vi "Main.vi"() -> ()   [LabVIEW 2011]
uses:
  VendingStateCtr.ctl
panel:
  out "결과":string
  out "현재 잔액":i32
  in  "종료 버튼":bool
  in  "환불":bool
  in  "콜라 구입":bool
  in  "500원 투입":bool
  in  "100원 투입":bool
  in  "50원 투입":bool
  in  "Enum":T1
  # "동전 투입 버튼"
  # "자판기 기능 버튼"
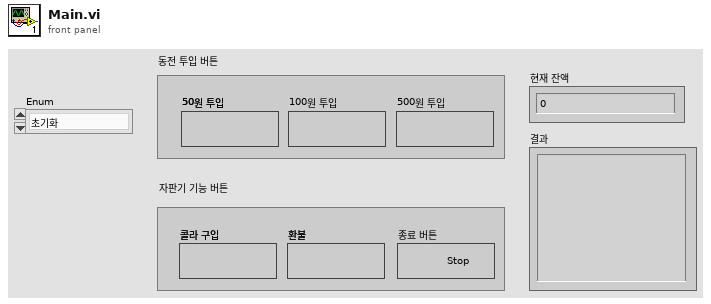
[diagram p1: front panel]
types:
  T1 = typedef "VendingStateCtr.ctl" = enum16{"초기화", "대기", "100원 투입", "500원 투입", "50원 투입", "판매", "환불", "종료"}
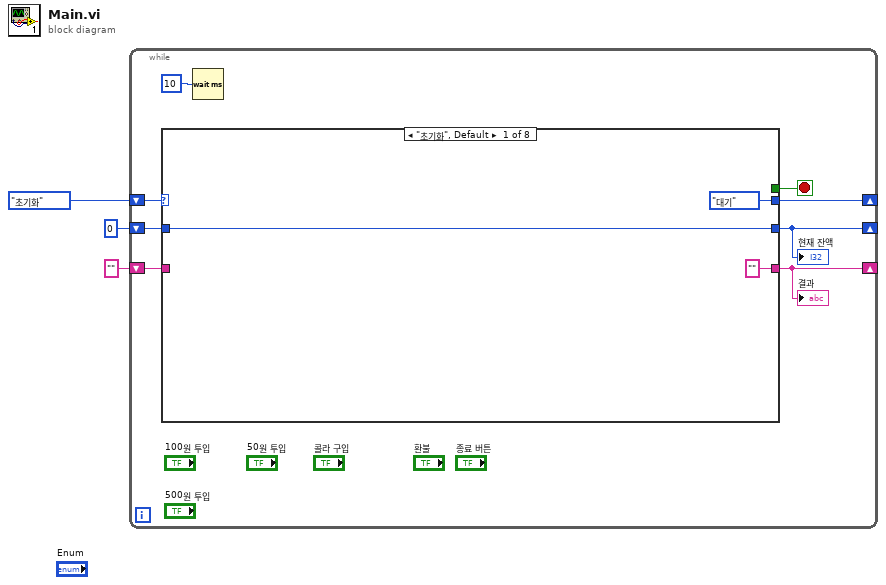
[diagram p0: block diagram]
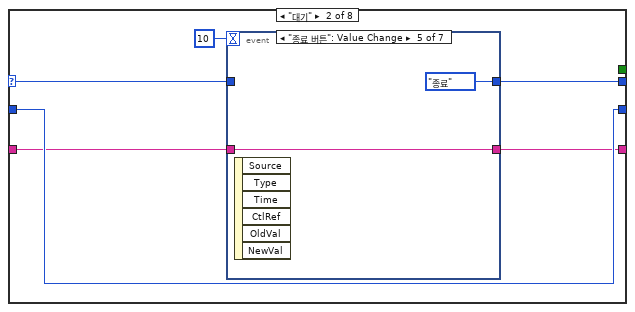
[diagram p2: hidden frame]
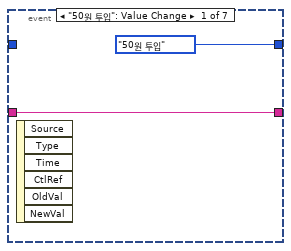
[diagram p3: hidden frame]
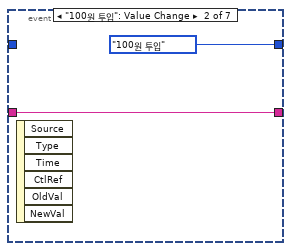
[diagram p4: hidden frame]
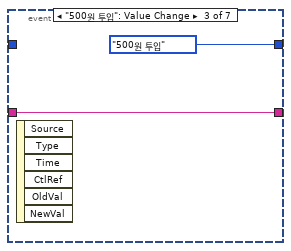
[diagram p5: hidden frame]
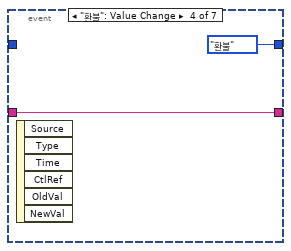
[diagram p6: hidden frame]
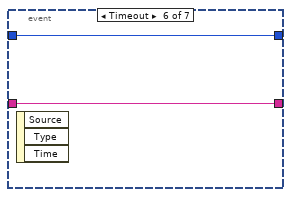
[diagram p7: hidden frame]
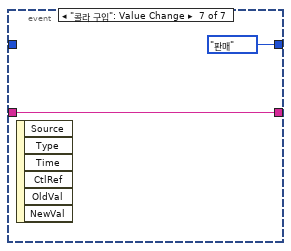
[diagram p8: hidden frame]
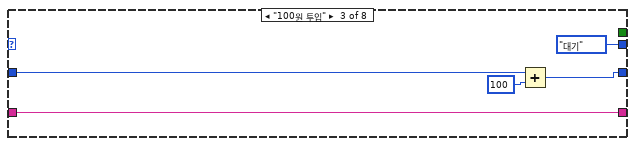
[diagram p9: hidden frame]
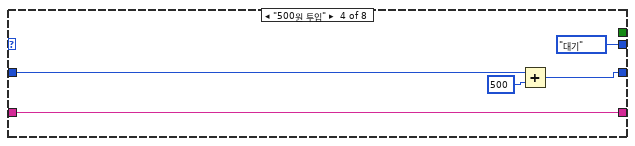
[diagram p10: hidden frame]
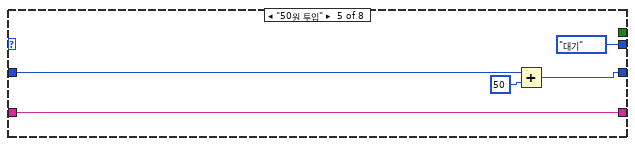
[diagram p11: hidden frame]
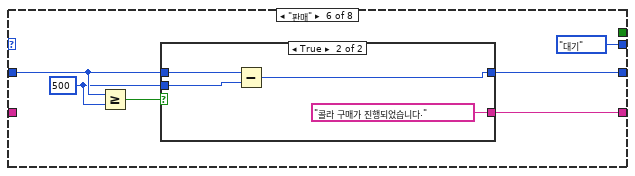
[diagram p12: hidden frame]
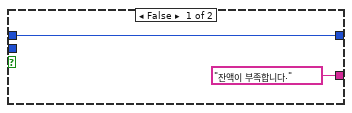
[diagram p13: hidden frame]
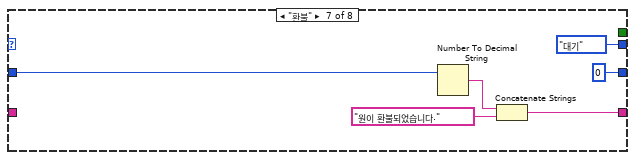
[diagram p14: hidden frame]
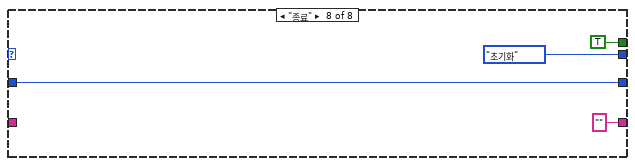
[diagram p15: hidden frame]
diagram:
  n1 = while {
    shift-right: [w9] -> _
    shift-left: VendingStateCtr."초기화" ("Enum") -> [w11]
    shift-right: [w7] -> _
    shift-left: 0 -> [w10]
    shift-right: [w4] -> _
    shift-left: "" -> [w5]
    stop <- w6 stop-if-true
    n2 = case shown="\"초기화\", Default" w11 {
      selector: w11 -> [_ w15 _ _ _ _ _ _]
      tunnel: w10 -> [w14 w18 w39 w44 w49 w52 w67 w70]
      tunnel: [w14 w18 w37 w42 w47 w51 0 w70] -> w7
      tunnel: [VendingStateCtr."대기" ("Enum") w19 VendingStateCtr."대기" ("Enum") VendingStateCtr."대기" ("Enum") VendingStateCtr."대기" ("Enum") VendingStateCtr."대기" ("Enum") VendingStateCtr."대기" ("Enum") VendingStateCtr."초기화" ("Enum")] -> w9
      tunnel: [_ _ _ _ _ _ _ TRUE] -> w6
      tunnel: ["" w17 w35 w40 w45 w53 w64 ""] -> w4
      tunnel: w5 -> [_ w16 w35 w40 w45 _ _ _]
      frame "초기화", Default {
      }
      frame "대기" {
        n3 = event shown="[4] \"종료 버튼\": Value Change" {
          selector: _ -> [_ _ _ _ _ _ _]
          dyn-events: _ -> [_ _ _ _ _ _ _]
          timeout: 10 -> [_ _ _ _ _ _ _]
          tunnel: [VendingStateCtr."50원 투입" ("Enum") VendingStateCtr."100원 투입" ("Enum") VendingStateCtr."500원 투입" ("Enum") VendingStateCtr."환불" ("Enum") VendingStateCtr."종료" ("Enum") w31 VendingStateCtr."판매" ("Enum")] -> w19
          tunnel: [w21 w23 w25 w27 w29 w32 w33] -> w17
          tunnel: w16 -> [w21 w23 w25 w27 w29 w32 w33]
          tunnel: w15 -> [_ _ _ _ _ w31 _]
          event "50원 투입": Value Change {
            n4 = event-data() -> ()  [unwired: 1 in, 6 out]
          }
          event "100원 투입": Value Change {
            n5 = event-data() -> ()  [unwired: 1 in, 6 out]
          }
          event "500원 투입": Value Change {
            n6 = event-data() -> ()  [unwired: 1 in, 6 out]
          }
          event "환불": Value Change {
            n7 = event-data() -> ()  [unwired: 1 in, 6 out]
          }
          event "종료 버튼": Value Change {
            n8 = event-data() -> ()  [unwired: 1 in, 6 out]
          }
          event Timeout {
            n9 = event-data() -> ()  [unwired: 1 in, 3 out]
          }
          event "콜라 구입": Value Change {
            n10 = event-data() -> ()  [unwired: 1 in, 6 out]
          }
        }
      }
      frame "100원 투입" {
        n11 = Add(x=w39, y=100) -> (x+y=w37:i32)
      }
      frame "500원 투입" {
        n12 = Add(x=w44, y=500) -> (x+y=w42:i32)
      }
      frame "50원 투입" {
        n13 = Add(x=w49, y=50) -> (x+y=w47:i32)
      }
      frame "판매" {
        w50 = 500 ("y")
        n14 = Greater Or Equal?(x=w52, y=w50) -> (x >= y?=w54:bool)
        n15 = case shown="True" w54 {
          tunnel: ["잔액이 부족합니다." "콜라 구매가 진행되었습니다."] -> w53
          tunnel: w52 -> [w56 w60]
          tunnel: [w56 w58] -> w51
          tunnel: w50 -> [_ w59]
          frame False {
          }
          frame True {
            n16 = Subtract(x=w60, y=w59) -> (x-y=w58:i32)
          }
        }
      }
      frame "환불" {
        n17 = Number To Decimal String(number=w67) -> (decimal integer string=w66:string)  [unwired: 1 in]
        n18 = Concatenate Strings(w66, "원이 환불되었습니다." ("string")) -> (w64:string)
      }
      frame "종료" {
      }
    }
    "현재 잔액" <- w7
    "결과" <- w4
    n19 = Wait (ms)(milliseconds to wait=u32 10) -> ()  [unwired: 1 out]
  }
